vi "_AllThings uPython.vi"   [LabVIEW 2016]
uses:
  uPythonX/uPythonX.xctl
  SystemLink/Systemlink Tag.xctl
  ColorText/Code.xctl
panel:
  # "CHeck Up arrow"
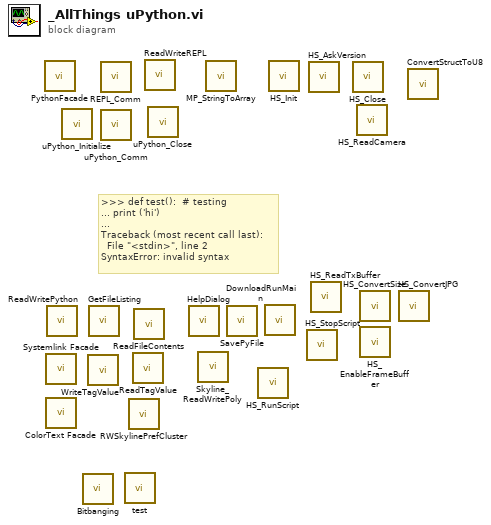
[diagram p0: block diagram]
diagram:
  # ">>> def test():  # testing\n... print ('hi')\n... \nTraceback (most recent call last):\n  File \"<stdin>\", line 2\nSyntaxError: invalid syntax"
  n1 = call "PythonFacade.vi"() -> ()  [unwired: 6 in, 3 out]
  n2 = call "Systemlink Facade.vi"() -> ()  [unwired: 6 in, 3 out]
  n3 = call "ColorText Facade.vi"() -> ()  [unwired: 6 in, 3 out]
  n4 = call "ReadWritePython.vi"() -> ()  [unwired: 6 in, 6 out]
  n5 = call "uPython_Initialize.vi"() -> ()  [unwired: 10 in, 2 out]
  n6 = call "Bitbanging.vi"() -> ()  [unwired: 12 in]
  n7 = call "WriteTagValue.vi"() -> ()  [unwired: 12 in]
  n8 = call "GetFileListing.vi"() -> ()  [unwired: 10 in, 2 out]
  n9 = call "REPL_Comm.vi"() -> ()  [unwired: 11 in, 1 out]
  n10 = call "uPython_Comm.vi"() -> ()  [unwired: 7 in, 5 out]
  n11 = call "test.vi"() -> ()  [unwired: 12 in]
  n12 = call "RWSkylinePrefCluster.vi"() -> ()  [unwired: 10 in, 2 out]
  n13 = call "ReadTagValue.vi"() -> ()  [unwired: 11 in, 1 out]
  n14 = call "ReadFileContents.vi"() -> ()  [unwired: 10 in, 2 out]
  n15 = call "ReadWriteREPL.vi"() -> ()  [unwired: 7 in, 5 out]
  n16 = call "uPython_Close.vi"() -> ()  [unwired: 11 in, 1 out]
  n17 = call "HelpDialog.vi"() -> ()  [unwired: 12 in]
  n18 = call-poly "Skyline_ReadWritePoly.vi"() -> ()  [unwired: 11 in, 1 out]
  n19 = call "MP_StringToArray.vi"() -> ()  [unwired: 11 in, 1 out]
  n20 = call "SavePyFile.vi"() -> ()  [unwired: 9 in, 3 out]
  n21 = call "HS_RunScript.vi"() -> ()  [unwired: 8 in, 4 out]
  n22 = call "DownloadRunMain.vi"() -> ()  [unwired: 9 in, 3 out]
  n23 = call "HS_Init.vi"() -> ()  [unwired: 10 in, 2 out]
  n24 = call "HS_StopScript.vi"() -> ()  [unwired: 8 in, 4 out]
  n25 = call "HS_AskVersion.vi"() -> ()  [unwired: 8 in, 4 out]
  n26 = call "HS_ReadTxBuffer.vi"() -> ()  [unwired: 8 in, 4 out]
  n27 = call "HS_Close.vi"() -> ()  [unwired: 12 in]
  n28 = call "HS_ReadCamera.vi"() -> ()  [unwired: 4 in, 8 out]
  n29 = call "HS_ConvertSize.vi"() -> ()  [unwired: 10 in, 2 out]
  n30 = call "HS_EnableFrameBuffer.vi"() -> ()  [unwired: 8 in, 4 out]
  n31 = call "HS_ConvertJPG.vi"() -> ()  [unwired: 10 in, 2 out]
  n32 = call "ConvertStructToU8.vi"() -> ()  [unwired: 1 in, 1 out]
